vi "Tophat Init LUT.vi"(7 "Number of  Elements":i32=80000, 8 "Df":i16=200, 9 "f0":i16=1350) -> (3 "Init Data Out":i16[](array[numeric]))   [LabVIEW 2015]
uses:
  <vilib>/Analysis/2dsp.llb/Inverse Real FFT.vi
  <vilib>/Analysis/NI_AALPro.lvlib
panel:
  out "f(t) half":i16[](graph)
  out "min value":i32=-32360
  out "max value":i32=-32768
  out "f(t)":i32[](graph)
  out "Frequency Domain Signal":i64[](graph)
  # "This is the max number of elements that will sit in a 16 bit wide block of memory"
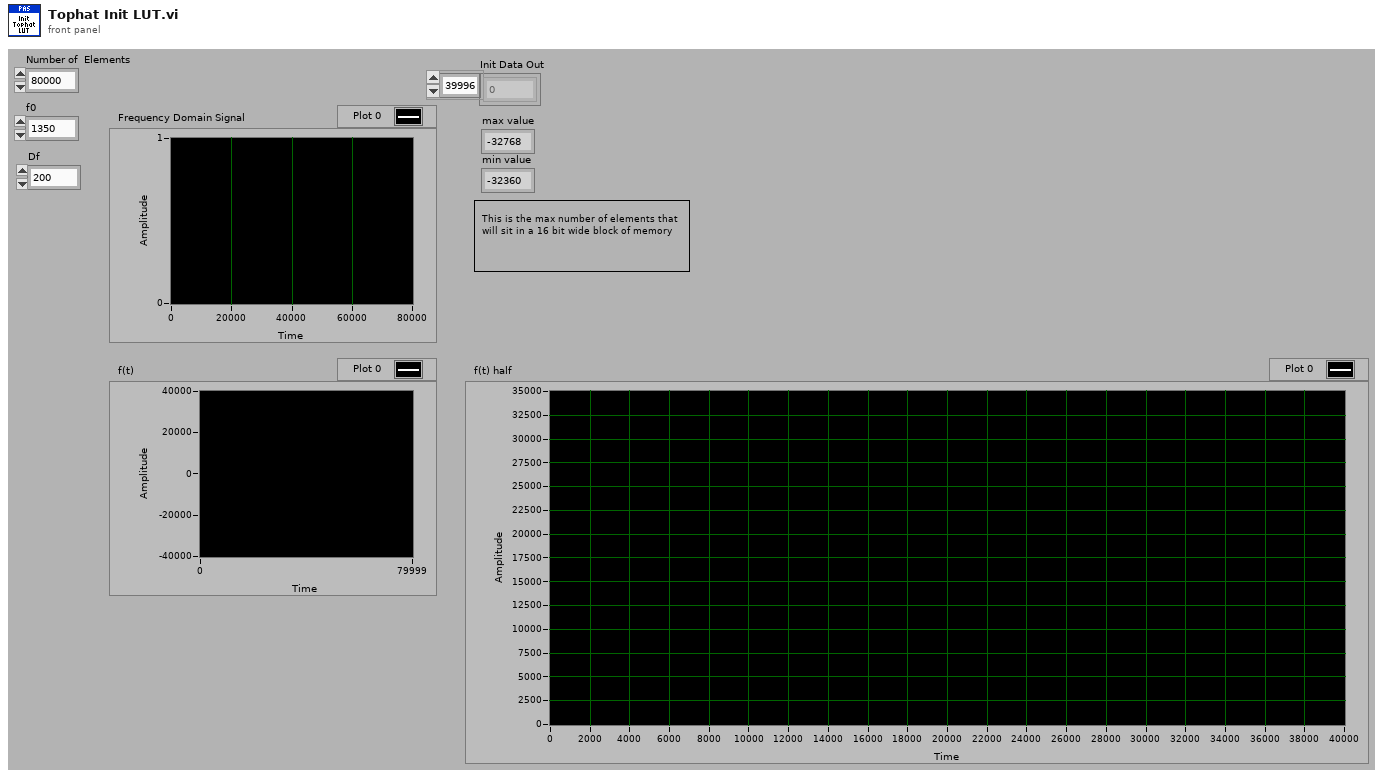
[diagram p1: front panel]
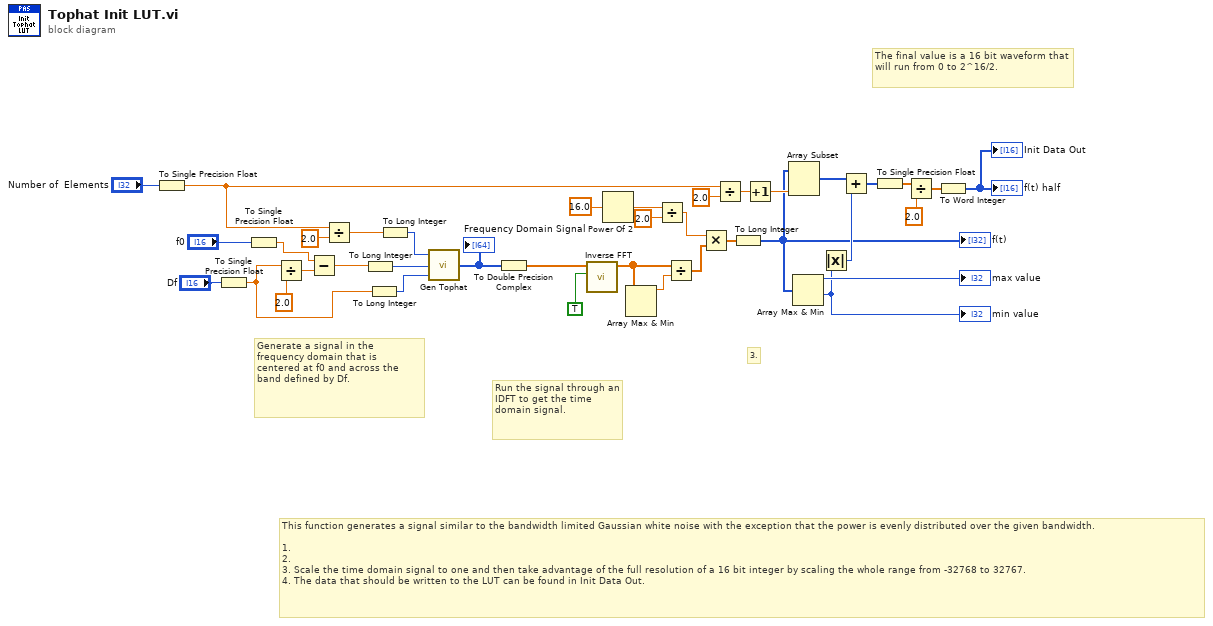
[diagram p0: block diagram]
diagram:
  # "The final value is a 16 bit waveform that will run from 0 to 2^16/2."
  # "Generate a signal in the frequency domain that is centered at f0 and across the band defined by Df."
  # "3."
  # "Run the signal through an IDFT to get the time domain signal."
  # "This function generates a signal similar to the bandwidth limited Gaussian white noise with the exception that the power is evenly distributed over the given bandwidth.\n\n1. \n2. \n3. Scale the time domain signal to one and then take advantage of the full resolution of a 16 bit integer by scaling the whole range from -32768 to 32767.\n4. The data that should be written to the LUT can be found in Init Data Out."
  n1 = To Single Precision Float(number="Number of  Elements") -> (single precision float=w9:sgl)
  n2 = To Single Precision Float(number="Df") -> (single precision float=w4:sgl)
  n3 = To Single Precision Float(number="f0") -> (single precision float=w11:sgl)
  n4 = Divide(x=w4, y=sgl 2.0) -> (x/y=w30:sgl)
  n5 = Subtract(x=w11, y=w30) -> (x-y=w6:sgl)
  n6 = Divide(x=w9, y=sgl 2.0) -> (x/y=w8:sgl)
  n7 = To Long Integer(number=w6) -> (32bit integer=w5:i32)
  n8 = To Long Integer(number=w4) -> (32bit integer=w3:i32)
  n9 = To Long Integer(number=w8) -> (32bit integer=w7:i32)
  n10 = call "Gen Tophat.vi"("Frequency Span"=w3, "Lower Frequency \nLocation"=w5, "Nyquist Frequency\nLocation"=w7) -> ("Waveform Graph"=w2:i64[])
  "Frequency Domain Signal" <- w2
  n11 = To Double Precision Complex(1:w2) -> (0:w1:cdb[])
  n12 = call-poly <vilib>:"Inverse FFT.vi"("shift?"=TRUE, "FFT {X}"=w1) -> ("X"=w34:dbl[])  [unwired: 9 out]
  n13 = Power Of 2(x=sgl 16.0) -> (2^x=w33:sgl)
  n14 = Array Max & Min(array=w34) -> (max value=w24:dbl)  [unwired: 3 out]
  n15 = Divide(x=w33, y=sgl 2.0) -> (x/y=w31:sgl)
  n16 = Divide(x=w34, y=w24) -> (x/y=w25:dbl[])
  n17 = Multiply(x=w31, y=w25) -> (x*y=w17:dbl[])
  n18 = Divide(x=w9, y=sgl 2.0) -> (x/y=w27:sgl)
  n19 = To Long Integer(number=w17) -> (32bit integer=w16:i32[])
  "f(t)" <- w16
  n20 = Increment(x=w27) -> (x+1=w26:sgl)
  n21 = Array Subset(array=w16, length=w26) -> (w23:i32[])  [unwired: 1 in]
  n22 = Array Max & Min(array=w16) -> (max value=→"max value":i32, min value=w19:i32)  [unwired: 2 out]
  "min value" <- w19
  n23 = Absolute Value(x=w19) -> (abs(x)=w18:i32)
  n24 = Add(x=w23, y=w18) -> (x+y=w15:i32[])
  n25 = To Single Precision Float(number=w15) -> (single precision float=w14:sgl[])
  n26 = Divide(x=w14, y=sgl 2.0) -> (x/y=w21:sgl[])
  n27 = To Word Integer(number=w21) -> (16bit integer=→"Init Data Out" →"f(t) half":i16[])
